vi "Set Calling VI Wnd Topmost &amp; Active.vi"(8 "Error In":errorcluster) -> (0 "Error Out":errorcluster)   [LabVIEW 2015, in "Win32 Util.lvlib"]
doc: "Sets the Caller VIs front panel Topmost (no other windows can be in front), Active (title bar is selected), and gives Focus (keystrokes are directed to the panel).\n\nCopyright © 2010 Blue Ridge Test, Inc.\nwww.BlueRidgeTest.com"
uses:
  LabSDL2/Source/Libraries/Win32 Util/Win32 Util.lvlib
  USER32.DLL
panel:
  out "Show\\Rest":i32
  out "Minimized?":i32
  out "FG hWnd":i32
  out "FG ProcID":i32
  out "hWnd ProcID":i32
  out "SetFG\\Attach":i32
  # "NP 2017-07-14\nTaken from\nhttps://lavag.org/topic/12751-how-do-you-make-your-application-window-frontmost/?do=findComment&comment=113072\n\nNot sure on copyright. Suspct this is public domain."
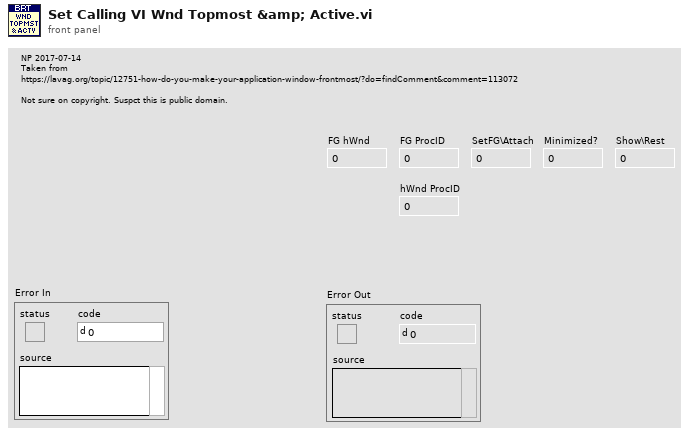
[diagram p1: front panel]
types:
  T1 = enum32{"Invalid", "Standard", "Closed", "Hidden", "Minimized", "Maximized"}
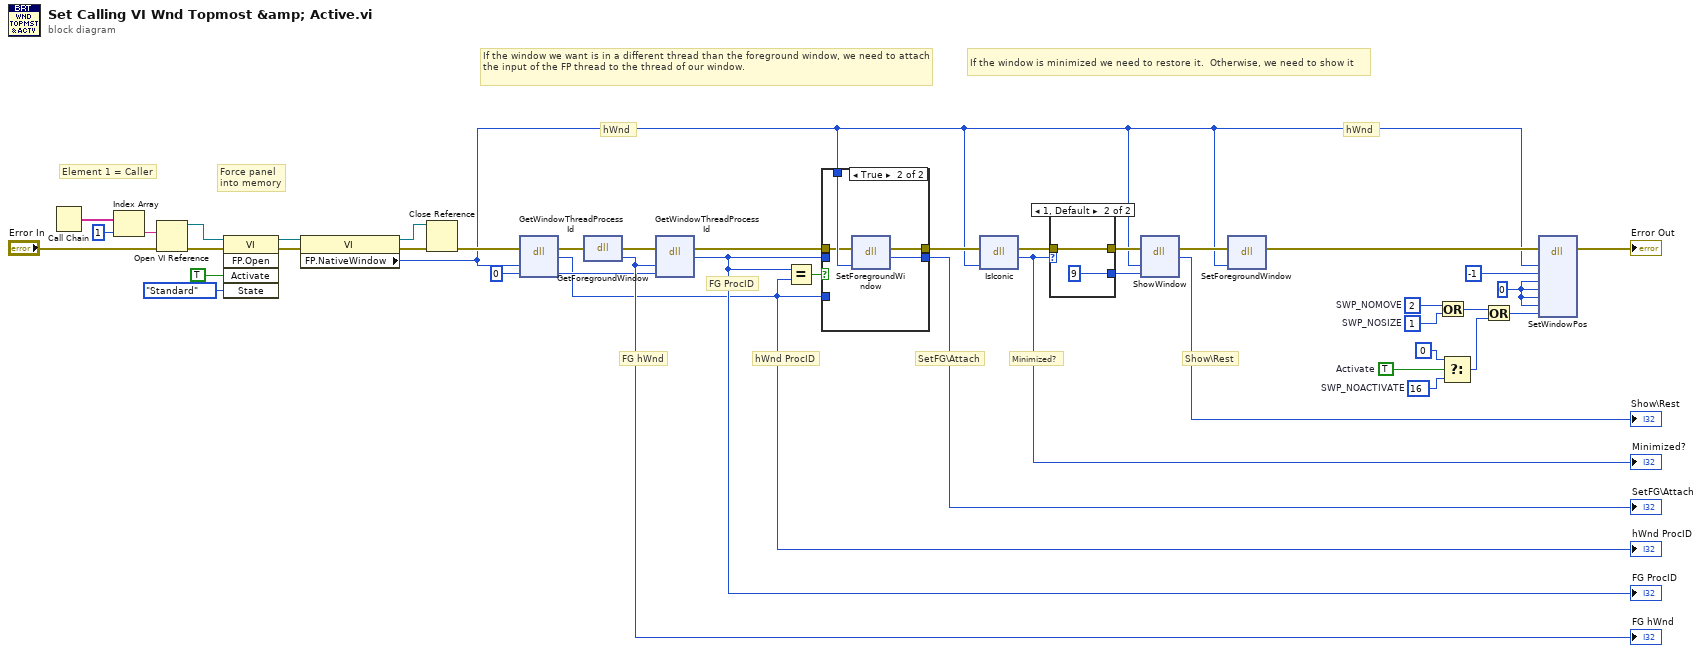
[diagram p0: block diagram]
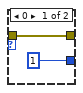
[diagram p2: hidden frame]
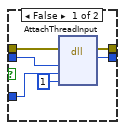
[diagram p3: hidden frame]
diagram:
  w19 = 0 ("lpdwProcessID")
  w32 = TRUE  # Activate
  w31 = u32 2  # SWP_NOMOVE
  w30 = u32 1  # SWP_NOSIZE
  w29 = u32 16  # SWP_NOACTIVATE
  w33 = 0
  # "hWnd ProcID"
  # "Show\\Rest"
  # "Minimized?"
  # "SetFG\\Attach"
  # "Force panel\ninto memory"
  # "FG hWnd"
  # "FG ProcID"
  # "hWnd"
  # "If the window is minimized we need to restore it.  Otherwise, we need to show it"
  # "hWnd"
  # "If the window we want is in a different thread than the foreground window, we need to attach the input of the FP thread to the thread of our window."
  # "Element 1 = Caller"
  n1 = Call Chain() -> (call chain=w39:string[])
  n2 = Index Array(array=w39, index=1) -> (element=w38:string)
  n3 = Open VI Reference(vi path=w38, error in (no error)="Error In") -> (vi reference=w35:refnum<vi>, error out=w36:errorcluster)  [unwired: 4 in]
  n4 = invoke class="VI" method="FP.Open"(reference=w35, error in=w36, "Activate"=TRUE ("Activate?"), "State"=T1."Standard") -> (reference out=w5:refnum<vi>, error out=w6:errorcluster)  [unwired: 1 in, 3 out]
  n5 = property class="VI"(reference=w5, error in=w6) -> (reference out=w3:refnum<vi>, error out=w4:errorcluster, "FP.NativeWindow"=w1:u64)
  n6 = Close Reference(reference=w3, error in (no error)=w4) -> (error out=w2:errorcluster)
  n7 = dll-call lib="user32" fn="GetWindowThreadProcessId" label="Get\nWindow\nThread\nProcess\nId"(error in=w2, "hWnd"=w1, "lpdwProcessID"=w19) -> (error out=w14:errorcluster, w13:i32)  [unwired: 4 in, 1 out]
  "hWnd ProcID" <- w13
  n8 = dll-call lib="user32" fn="GetForegroundWindow" label="Get\nForeground\nWindow"(error in=w14) -> (error out=w15:errorcluster, "hWnd"=w20:i32)  [unwired: 2 in, 1 out]
  "FG hWnd" <- w20
  n9 = dll-call lib="user32" fn="GetWindowThreadProcessId" label="Get\nWindow\nThread\nProcess\nId"(error in=w15, "hWnd"=w20, "lpdwProcessID"=w19) -> (error out=w12:errorcluster, w17:i32)  [unwired: 4 in, 1 out]
  "FG ProcID" <- w17
  n10 = Equal?(x=w17, y=w13) -> (x = y?=w18:bool)
  n11 = case shown="True" w18 {
    tunnel: w17 -> [w48 _]
    tunnel: w13 -> [w47 _]
    tunnel: w1 -> [_ w52]
    tunnel: [w45 w51] -> w16
    tunnel: w12 -> [w44 w50]
    tunnel: [w43 w49] -> w23
    frame False {
      n12 = dll-call lib="user32" fn="AttachThreadInput" label="Attach\nThread\nInput"(error in=w44, "idAttach"=w48, "idAttachTo"=w47, "fAttach"=1) -> (error out=w43:errorcluster, w45:i32)  [unwired: 5 in, 1 out]
    }
    frame True {
      n13 = dll-call lib="user32" fn="SetForegroundWindow" label="Set\nForeground\nWindow"(error in=w50, "hWnd"=w52) -> (error out=w49:errorcluster, w51:i32)  [unwired: 3 in, 1 out]
    }
  }
  "SetFG\\Attach" <- w16
  n14 = dll-call lib="user32" fn="IsIconic"(error in=w23, "hWnd"=w1) -> (error out=w7:errorcluster, w11:i32)  [unwired: 3 in, 1 out]
  "Minimized?" <- w11
  n15 = case shown="1, Default" w11 {
    tunnel: [i16 1 ("nCmdshow") i16 9 ("nCmdshow")] -> w10
    tunnel: [w53 w55] -> w8
    tunnel: w7 -> [w53 w55]
    frame 0 {
    }
    frame 1, Default {
    }
  }
  n16 = dll-call lib="user32.dll" fn="ShowWindow"(error in=w8, "hWnd"=w1, "nCmdshow"=w10) -> (error out=w22:errorcluster, →"Show\\Rest":i32)  [unwired: 4 in, 1 out]
  n17 = dll-call lib="user32" fn="SetForegroundWindow" label="Set\nForeground\nWindow"(error in=w22, "hWnd"=w1) -> (error out=w21:errorcluster)  [unwired: 4 in, 1 out]
  n18 = Or(x=w31, y=w30) -> (x .or. y?=w26:u32)
  n19 = Select(t=u32 0, s=w32, f=w29) -> (s? t:f=w27:u32)
  n20 = Or(x=w26, y=w27) -> (x .or. y?=w25:u32)
  n21 = dll-call lib="USER32.DLL" fn="SetWindowPos"(error in=w21, "hWnd"=w1, "hWndInsertAfter"=-1, "left"=w33, "top"=w33, "width"=w33, "height"=w33, "fuFlags"=w25) -> (error out=→"Error Out":errorcluster)  [unwired: 8 in, 3 out]
